vi "Set Relay State.vi"(4 "State":bool, 6 "Relay Name":string, 8 "error in (no error)":errorcluster, 9 "nodePath":string, 10 "NIVS.System Definition Root":refnum<k24>, 11 "WorkspaceManager in":T1) -> (0 "error out":errorcluster, 3 "WorkspaceManager out":T1)   [LabVIEW 2013]
uses:
  NationalInstruments.VeriStand.SystemStorage
  <vilib>/NI Veristand/Execution/Workspace/WorkspaceAPI.ctl
  NationalInstruments.VeriStand.ClientAPI
  NationalInstruments.VeriStand
  <vilib>/NI Veristand/Execution/Workspace/NI VeriStand - Set Single Channel Value.vi
  <vilib>/NI Veristand/Execution/Workspace/NI_VS Workspace ExecutionAPI.lvlib
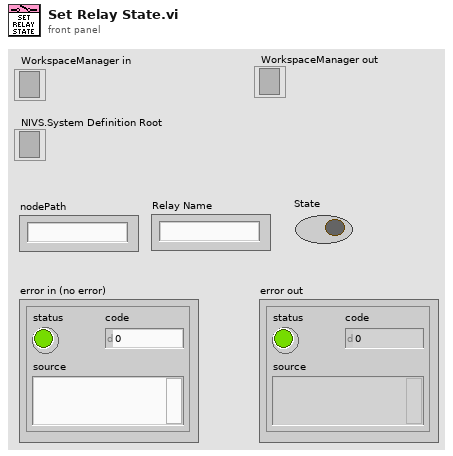
[diagram p1: front panel]
types:
  T1 = typedef "NI_VS Workspace ExecutionAPI.lvlib/WorkspaceAPI.ctl" = refnum<k24>
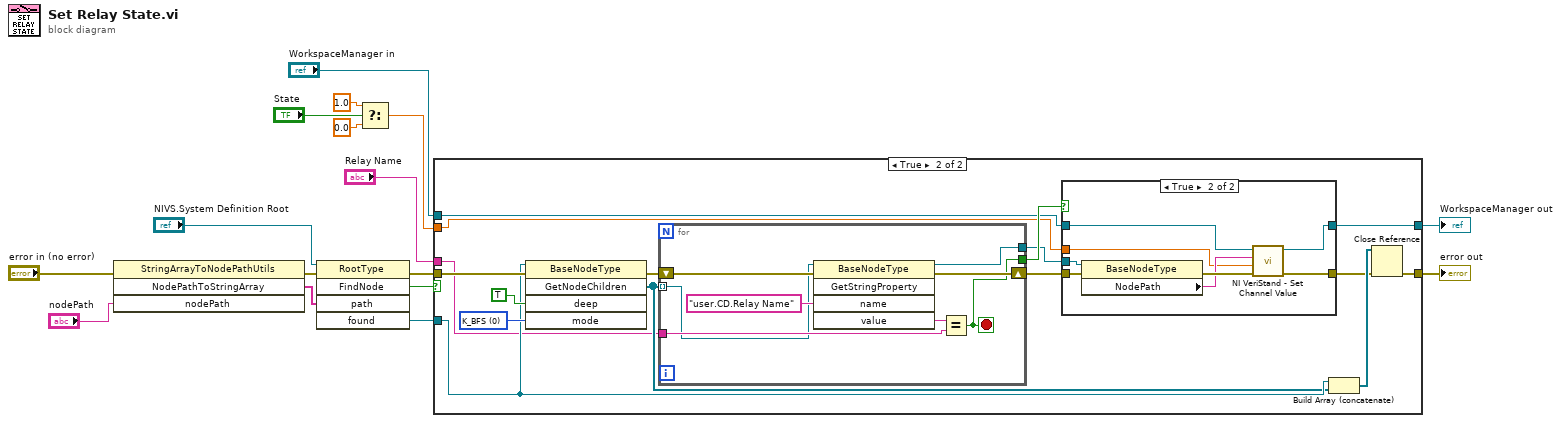
[diagram p0: block diagram]
diagram:
  n1 = invoke class="StringArrayToNodePathUtils" method="NodePathToStringArray"(error in="error in (no error)", "nodePath"="nodePath") -> (error out=w15:errorcluster, "NodePathToStringArray"=w16:string[])  [unwired: 2 in, 2 out]
  n2 = invoke class="RootType" method="FindNode"(reference="NIVS.System Definition Root", error in=w15, "path"=w16) -> (error out=w14:errorcluster, "FindNode"=w11:bool, "found"=w10:refnum<k24>)  [unwired: 2 in, 2 out]
  n3 = Select(t=1.0, s="State", f=0.0) -> (s? t:f=w1:dbl)
  n4 = case shown="True" w11 {
    tunnel: w14 -> [w18 w34]
    tunnel: w10 -> [_ w29]
    tunnel: "WorkspaceManager in" -> [w17 w21]
    tunnel: [w17 w20] -> w8
    tunnel: [w18 w30] -> w7
    tunnel: "Relay Name" -> [_ w26]
    tunnel: w1 -> [_ w19]
    frame False {
    }
    frame True {
      w32 = 0 items=["K_BFS", "K_DFS", "K_CHILDONLY", "K_UP"] ("mode")
      n5 = invoke class="BaseNodeType" method="GetNodeChildren"(reference=w29, error in=w34, "deep"=TRUE, "mode"=w32) -> (error out=w31:errorcluster, "GetNodeChildren"=w28:refnum<k24>[])  [unwired: 1 in, 3 out]
      n6 = for {
        tunnel: w28 -> [w46] mode=indexing
        shift-right: [w49] -> w25
        shift-left: w31 -> [w47]
        tunnel: w26 -> [w51]
        tunnel: [w48] -> w22
        tunnel: [w45] -> w23
        stop <- w45 stop-if-true
        n7 = invoke class="BaseNodeType" method="GetStringProperty"(reference=w46, error in=w47, "name"="user.CD.Relay Name") -> (reference out=w48:refnum<k24>, error out=w49:errorcluster, "value"=w50:string)  [unwired: 2 in, 2 out]
        n8 = Equal?(x=w50, y=w51) -> (x = y?=w45:bool)
      }
      n9 = case shown="True" w23 {
        tunnel: w25 -> [w36 w43]
        tunnel: [w36 w44] -> w24
        tunnel: w22 -> [_ w42]
        tunnel: w21 -> [w35 w39]
        tunnel: [w35 w38] -> w20
        tunnel: w19 -> [_ w37]
        frame False {
        }
        frame True {
          n10 = property class="BaseNodeType"(reference=w42, error in=w43) -> (error out=w41:errorcluster, "NodePath"=w40:string)  [unwired: 1 out]
          n11 = call-poly <vilib>:"NI VeriStand - Set Channel Value.vi"("error in (no error)"=w41, "Value"=w37, "Channel"=w40, "WorkspaceManager in"=w39) -> ("error out"=w44:errorcluster, "WorkspaceManager out"=w38:T1)  [unwired: 6 in]
        }
      }
      n12 = Build Array (concatenate)(w29, w28) -> (w27:refnum<k24>[])
      n13 = Close Reference(reference=w27, error in (no error)=w24) -> (error out=w30:errorcluster)
    }
  }
  "WorkspaceManager out" <- w8
  "error out" <- w7
